vi "FPGA_NIFPGAInterfaceFPGAResourceConstant.vi"() -> (0 "NumberOfRelays":u32=4, 1 "NumberOfPWMs":u32=20, 2 "NumberOfEncoders":u32=8, 3 "NumberOfCounters":u32=8, 4 "NumberOfDIOOnboard":u32=10, 5 "NumberOfAIChannels":u8=8, 6 "NumberOfAnalogTriggers":u32=8, 7 "NumberOfInterrupts":u32=8, 8 "NumberOfAOChannels":u8=2, 9 "NumberOfSPI":i32=5, 11 "NumberOfSharedMXPpins":u32=16)   [LabVIEW 2017]
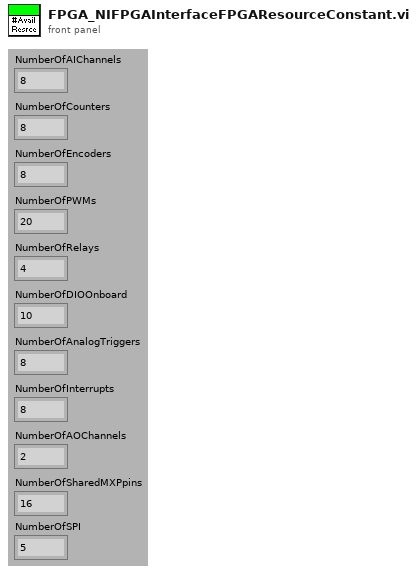
[diagram p1: front panel]
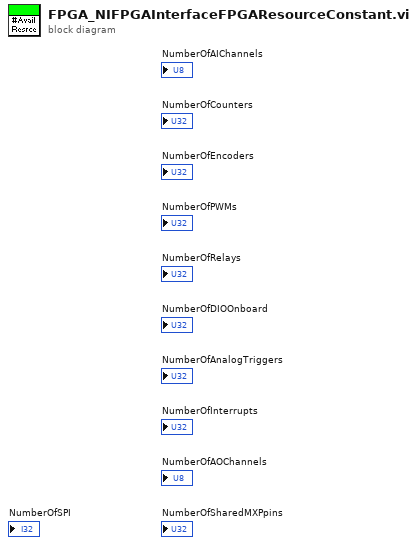
[diagram p0: block diagram]
diagram:
